vi "Source.Write.Scalar.Base10 (U16).vi"(9 "offset":i32, 10 "value":u16, 11 "error in":errorcluster) -> (1 "new offset":i32, 3 "error out":errorcluster)   [LabVIEW 2016, in "Memory Manager.lvlib" / "Static Error Handling.lvlib"]
doc: "Converts <b>value</b> into an decimal-formatted string, and writes the string to the <b>error in</b> source buffer at the specified <b>offset</b>."
uses:
  Static Error Handling.lvlib
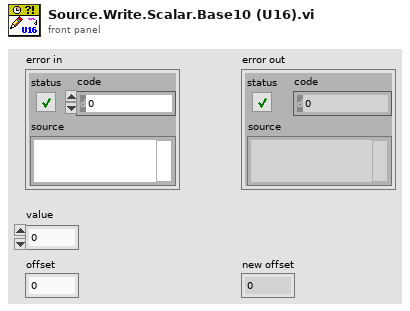
[diagram p1: front panel]
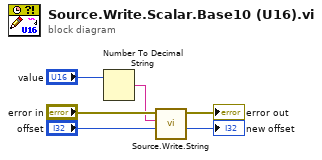
[diagram p0: block diagram]
diagram:
  n1 = Number To Decimal String(number="value") -> (decimal integer string=w2:string)  [unwired: 1 in]
  n2 = call "Source.Write.String.vi"("offset"="offset", "string"=w2, "error in"="error in") -> ("new offset"=→"new offset":i32, "error out"=→"error out":errorcluster)  [unwired: 7 in]
